vi "TESTE DA MASSA.vi"() -> ()   [LabVIEW 2019]
panel:
  in  "stop":bool
  in  "Offset":dbl min=-10.0 max=10.0
  in  "Amplitude":dbl min=0.0 max=10.0
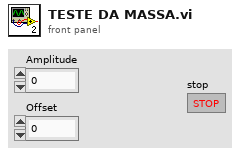
[diagram p1: front panel]
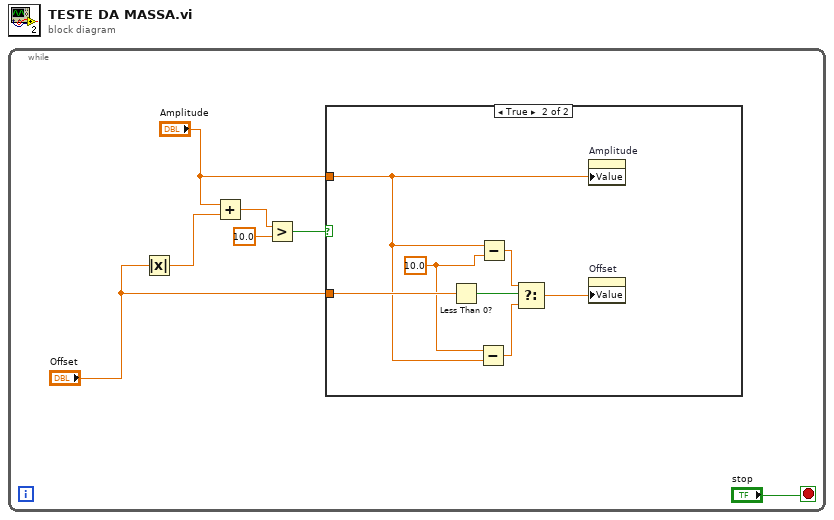
[diagram p0: block diagram]
diagram:
  n1 = while {
    stop <- "stop" stop-if-true
    n2 = Absolute Value(x="Offset") -> (abs(x)=w4:dbl)
    n3 = Add(x="Amplitude", y=w4) -> (x+y=w6:dbl)
    n4 = Greater?(x=w6, y=10.0) -> (0:w5:bool)
    n5 = case shown="True" w5 {
      tunnel: "Amplitude" -> [_ w9]
      tunnel: "Offset" -> [_ w14]
      frame False {
      }
      frame True {
        w10 = 10.0 ("y")
        n6 = Less Than 0?(x=w14) -> (x < 0?=w13:bool)
        n7 = Subtract(x=w10, y=w9) -> (x-y=w12:dbl)
        n8 = Subtract(x=w9, y=w10) -> (x-y=w11:dbl)
        n9 = Select(t=w11, s=w13, f=w12) -> (s? t:f=w8:dbl)
        n10 = property on="Amplitude" class="DigNum (strict)"("Value"=w9) -> ()  [unwired: 2 in, 2 out]
        n11 = property on="Offset" class="DigNum (strict)"("Value"=w8) -> ()  [unwired: 2 in, 2 out]
      }
    }
  }
